vi "Run Bfr Tx - Untimed.vi"(7 "Process in":refnum<class "Process.lvclass">, 8 "error in (no error)":errorcluster, 11 "Tx Loop Data in":T1={"General Resources"={"Packet Name"="", "Packet ID"=0, "Local IP Address"="", "Local Port"=0, "Multicast"=FALSE, "Multicast IP Address"=0, "Header Info"=[], "Byte Order"=enum."big-endian, network order", "Channel Data Types"=[], "Duplex Packets"=refnum}, "Header Details"={"Packet Size"=0, "Protocol Revision"=0, "System Definition Version"=0, "Source Node Name"="", "Packet ID"=0, "Number of Channels"=0, "Static Header Size"=0, "Total Header Size"=0}, "Buffer Resources"={"Data Buffer"=0, "Pointer Encoding"=enum."Direct Encoding", "Buffer Size"=0, "Raw Buffer Data"=[], "Is Buffered"=FALSE, "External Buffer"=FALSE, "Prepend Header"=FALSE, "Valid Buffer"=FALSE}, "Runtime Resources"={"Connection ID"=refnum, "Transmit Option"=enum."Always", "Destination IP Address"=0, "Destination Port"=0, "Multicast IP Address"=0, "TTL"=0, "Multicast"=FALSE, "Port as Channel"=FALSE, "ExecutionConfig"={"Loop Period"=0, "RT Loop Period"=-2, "Untimed Period"=0, "Target Processor"=0, "Priority"=0, "Thread Management"=enum."Untimed (Default)"}}, "Echo Resources"={"Transmit Echo Option"=enum."PCL Reset", "Packet Count"=0.0, "Counter Increment"=0.0, "Transmit Values"=[]}, "Buffer Option Support"={"Buffer Option"=enum."Static Buffer", "Sim Option"=enum."No Simulation"}, "Channel Resources"={"Transmit Flag"=refnum, "Transmit Echo"=refnum, "Transmit Bytes"=refnum, "Port Channel"=refnum, "Buffer (External)"=refnum, "Buffer (Local)"=refnum, "Timestamp"=refnum}, "Debug Resources"={"Debug Mode"=FALSE, "Debug Log File"=refnum, "Packet Name"=""}} {"Buffer Resources"."Data Buffer" format="%016x"}) -> (3 "Tx Loop Data out":T1={"General Resources"={"Packet Name"="", "Packet ID"=0, "Local IP Address"="", "Local Port"=0, "Multicast"=FALSE, "Multicast IP Address"=0, "Header Info"=[], "Byte Order"=enum."big-endian, network order", "Channel Data Types"=[], "Duplex Packets"=refnum}, "Header Details"={"Packet Size"=0, "Protocol Revision"=0, "System Definition Version"=0, "Source Node Name"="", "Packet ID"=0, "Number of Channels"=0, "Static Header Size"=0, "Total Header Size"=0}, "Buffer Resources"={"Data Buffer"=0, "Pointer Encoding"=enum."Direct Encoding", "Buffer Size"=0, "Raw Buffer Data"=[], "Is Buffered"=FALSE, "External Buffer"=FALSE, "Prepend Header"=FALSE, "Valid Buffer"=FALSE}, "Runtime Resources"={"Connection ID"=refnum, "Transmit Option"=enum."Always", "Destination IP Address"=0, "Destination Port"=0, "Multicast IP Address"=0, "TTL"=0, "Multicast"=FALSE, "Port as Channel"=FALSE, "ExecutionConfig"={"Loop Period"=0, "RT Loop Period"=-2, "Untimed Period"=0, "Target Processor"=0, "Priority"=0, "Thread Management"=enum."Untimed (Default)"}}, "Echo Resources"={"Transmit Echo Option"=enum."PCL Reset", "Packet Count"=0.0, "Counter Increment"=0.0, "Transmit Values"=[]}, "Buffer Option Support"={"Buffer Option"=enum."Static Buffer", "Sim Option"=enum."No Simulation"}, "Channel Resources"={"Transmit Flag"=refnum, "Transmit Echo"=refnum, "Transmit Bytes"=refnum, "Port Channel"=refnum, "Buffer (External)"=refnum, "Buffer (Local)"=refnum, "Timestamp"=refnum}, "Debug Resources"={"Debug Mode"=FALSE, "Debug Log File"=refnum, "Packet Name"=""}} {"Buffer Resources"."Data Buffer" format="%016x"})   [LabVIEW 2016, in "UDP-Custom-Device Engine.lvlib"]
uses:
  UDP-Custom-Device Engine.lvlib
  <vilib>/NI/NIVS Inline Async API/_VS Inline Async API/Process/Process.lvclass
  Types/Engine - Buffered Tx Loop Data.ctl
  Types/Engine - General Resources.ctl
  <vilib>/NI Veristand/VeriStand Data/Typedefs/Typedefs.Data Types.ctl
  Shared/Types/Shared - Duplex Settings.ctl
  Shared/Types/Shared - Header Details.ctl
  Types/Engine - Buffer Resources.ctl
  Shared/Types/Shared - Pointer Encoding.ctl
  Types/Engine - Tx Runtime Resources.ctl
  Shared/Types/Shared - Transmit Flag Options.ctl
  Types/Engine - Execution Config.ctl
  Shared/Types/Shared - Thread Management.ctl
  Types/Engine - Tx Echo Resources.ctl
  Shared/Types/Shared - Transmit Echo Options.ctl
  Types/Engine - Buffered Tx Buffer Option Support.ctl
  Shared/Types/Shared - Transmit Buffer Options.ctl
  Shared/Types/Shared - Transmit Sim Options.ctl
  Types/Engine - Buffered Tx Channel Refs.ctl
  <vilib>/NI/NIVS Inline Async API/_Data Access Engine/Data Access Engine/Types/Read.DVR.ctl
  <vilib>/NI/NIVS Inline Async API/_Data Access Engine/Access Type Classes/Read/Read.lvclass
  <vilib>/NI/NIVS Inline Async API/_Data Access Engine/Data Access Engine/Types/Write.DVR.ctl
  <vilib>/NI/NIVS Inline Async API/_Data Access Engine/Access Type Classes/Write/Write.lvclass
  Types/Engine - Debug Resources.ctl
  <vilib>/NI/NIVS Inline Async API/_Data Access Engine/Access Type Classes/Read/Read.lvclass/Read.ctl
  <vilib>/NI/NIVS Inline Async API/_Data Access Engine/Access Type Classes/Write/Write.lvclass/Write.ctl
  <vilib>/NI/NIVS Inline Async API/_VS Inline Async API/Process/Process.lvclass/Process.ctl
  <vilib>/NI Veristand/VeriStand Data/Pointer Operations/Pointer.Write.vi
  <vilib>/NI Veristand/VeriStand Data/Pointer Operations/Pointer.Write (String).vi
  <vilib>/NI Veristand/VeriStand Data/Pointer Operations/Pointer.Write (1D U8).vi
  <vilib>/NI Veristand/VeriStand Data/Pointer Operations/Pointer.Write (I32).vi
  <vilib>/NI Veristand/VeriStand Data/Pointer Operations/Pointer.Write (U16).vi
  <vilib>/NI/NIVS Inline Async API/_Data Access Engine/Data Access Engine/Methods/Data.Processes.Execute.vi
  <vilib>/NI/NIVS Inline Async API/_Data Access Engine/Data Access Engine/Methods/Read.Data.vi
  Transmit/Run Tx - Handle Transmit Option.vi
  Run Bfr Tx - Handle Transmit Size.vi
  Transmit/Run Tx - Handle Port Tx Check.vi
  <vilib>/NI/NIVS Inline Async API/_Data Access Engine/Data Access Engine/Methods/Write.Data.vi
  <vilib>/NI Veristand/VeriStand Data/Pointer Operations/Pointer.In-Place Read.vi
  <vilib>/NI Veristand/VeriStand Data/Pointer Operations/Pointer.In-Place Read (1D U8).vi
  Run Bfr Tx - FIFO Entry Size.vi
  Run Bfr Tx - FIFO Payload.vi
  Run Bfr Tx - FIFO Count Packets.vi
  Run Bfr Tx - FIFO Port.vi
  <vilib>/NI/NIVS Inline Async API/_VS Inline Async API/Error Handling Process/SubVIs/Error.ConvertArray.vi
  <vilib>/NI/NIVS Inline Async API/_Data Access Engine/Access Type Classes/Read/Read.ProcessData.vi
  <vilib>/NI Veristand/VeriStand Data/Type Conversion/Type Conversion.From Double.vi
  <vilib>/NI Veristand/VeriStand Data/Type Conversion/Type Conversion.From Double (I32).vi
  <vilib>/NI/NIVS Inline Async API/_Data Access Engine/Access Type Classes/Write/Write.ProcessData.vi
  <vilib>/NI Veristand/VeriStand Data/Pointer Operations/Pointer.Read.vi
  <vilib>/NI Veristand/VeriStand Data/Pointer Operations/Pointer.Read (I32).vi
  <vilib>/NI Veristand/VeriStand Data/Pointer Operations/Pointer.Read (U16).vi
  <vilib>/NI Veristand/VeriStand Data/Pointer Operations/Pointer.In-Place Read (I32).vi
  <vilib>/NI Veristand/VeriStand Data/Pointer Operations/Pointer.In-Place Read (U16).vi
  <vilib>/NI Veristand/VeriStand Data/VeriStand Data.lvlib
  Shared/UDP-Custom-Device Shared.lvlib
  <vilib>/NI/NIVS Inline Async API/_Data Access Engine/Data Access Engine/Data Access Engine.lvclass
panel:
  out "dataBuffer":u64 format="%016x"
  out "Tx Packet":string
  # "BUFFERED TRANSMIT\n- UNTIMED\n- ALL TARGETS"
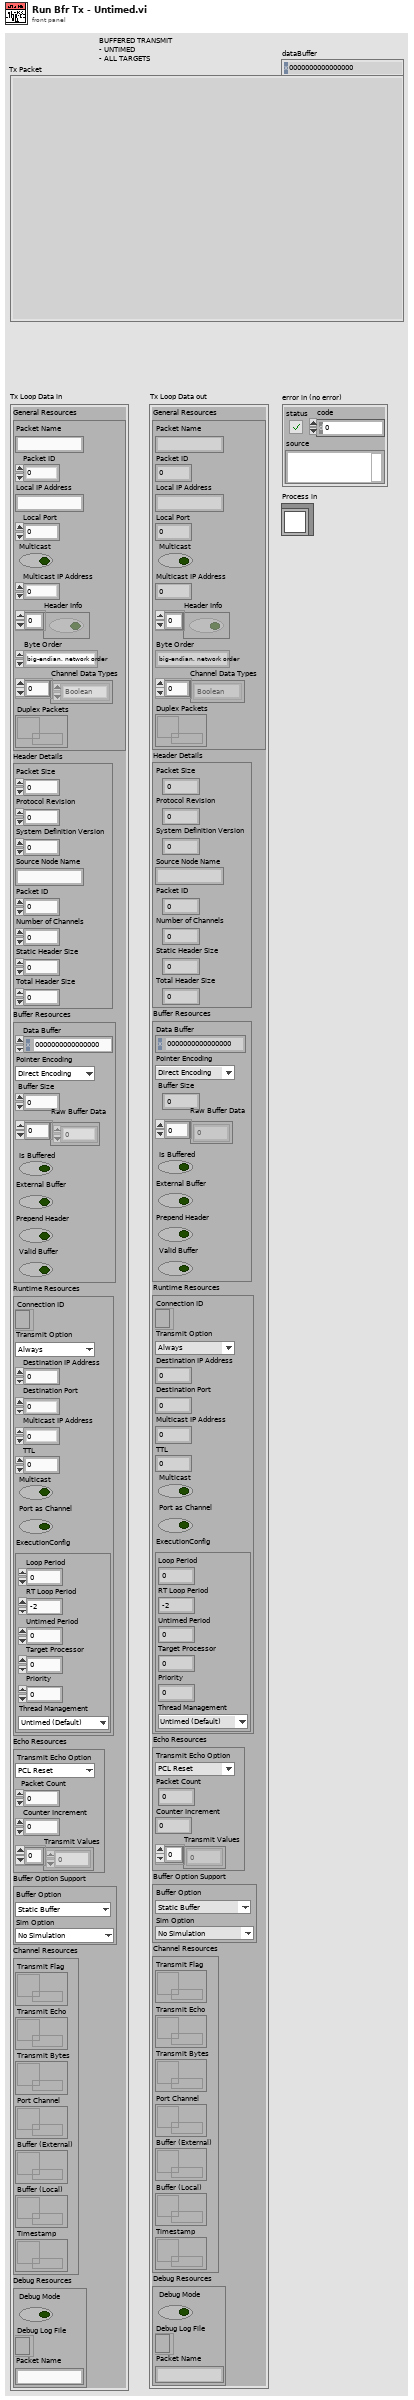
[diagram p1: front panel]
types:
  T1 = typedef "UDP-Custom-Device Engine.lvlib/Engine - Buffered Tx Loop Data.ctl" = cluster{"General Resources":T2, "Header Details":T4, "Buffer Resources":T5, "Runtime Resources":T7, "Echo Resources":T11, "Buffer Option Support":T13, "Channel Resources":T16, "Debug Resources":T19}
  T2 = typedef "UDP-Custom-Device Engine.lvlib/Engine - General Resources.ctl" = cluster{"Packet Name":string, "Packet ID":i32, "Local IP Address":string, "Local Port":i32, "Multicast":bool, "Multicast IP Address":u32, "Header Info":bool[], "Byte Order":enum16{"big-endian, network order", "native, host order", "little-endian"}, "Channel Data Types":T3[], "Duplex Packets":refnum<data-value>}
  T3 = typedef "VeriStand Data.lvlib/Typedefs.Data Types.ctl" = enum16{"Boolean", "Single", "Double", "I8", "I16", "I32", "I64", "U8", "U16", "U32", "U64"}
  T4 = typedef "UDP-Custom-Device Shared.lvlib/Shared - Header Details.ctl" = cluster{"Packet Size":u16, "Protocol Revision":u8, "System Definition Version":u64, "Source Node Name":string, "Packet ID":u32, "Number of Channels":u32, "Static Header Size":u16, "Total Header Size":u16}
  T5 = typedef "UDP-Custom-Device Engine.lvlib/Engine - Buffer Resources.ctl" = cluster{"Data Buffer":u64, "Pointer Encoding":T6, "Buffer Size":u64, "Raw Buffer Data":u8[], "Is Buffered":bool, "External Buffer":bool, "Prepend Header":bool, "Valid Buffer":bool}
  T6 = typedef "UDP-Custom-Device Shared.lvlib/Shared - Pointer Encoding.ctl" = enum16{"Direct Encoding", "Conversion Encoding"}
  T7 = typedef "UDP-Custom-Device Engine.lvlib/Engine - Tx Runtime Resources.ctl" = cluster{"Connection ID":refnum<k16>, "Transmit Option":T8, "Destination IP Address":u32, "Destination Port":u16, "Multicast IP Address":u32, "TTL":u16, "Multicast":bool, "Port as Channel":bool, "ExecutionConfig":T9}
  T8 = typedef "UDP-Custom-Device Shared.lvlib/Shared - Transmit Flag Options.ctl" = enum16{"Always", "One-Shot", "Toggle"}
  T9 = typedef "UDP-Custom-Device Engine.lvlib/Engine - Execution Config.ctl" = cluster{"Loop Period":i64, "RT Loop Period":i64, "Untimed Period":u32, "Target Processor":i32, "Priority":i32, "Thread Management":T10}
  T10 = typedef "UDP-Custom-Device Shared.lvlib/Shared - Thread Management.ctl" = enum16{"Untimed (Default)", "Timed (High Priority)"}
  T11 = typedef "UDP-Custom-Device Engine.lvlib/Engine - Tx Echo Resources.ctl" = cluster{"Transmit Echo Option":T12, "Packet Count":dbl, "Counter Increment":dbl, "Transmit Values":dbl[]}
  T12 = typedef "UDP-Custom-Device Shared.lvlib/Shared - Transmit Echo Options.ctl" = enum16{"PCL Reset", "Counter", "Mirror"}
  T13 = typedef "UDP-Custom-Device Engine.lvlib/Engine - Buffered Tx Buffer Option Support.ctl" = cluster{"Buffer Option":T14, "Sim Option":T15}
  T14 = typedef "UDP-Custom-Device Shared.lvlib/Shared - Transmit Buffer Options.ctl" = enum16{"Static Buffer", "FIFO Buffer", "FIFO Buffer + Port"}
  T15 = typedef "UDP-Custom-Device Shared.lvlib/Shared - Transmit Sim Options.ctl" = enum16{"No Simulation", "Counter", "Full Buffer", "FIFO Test", "FIFO + Port Test"}
  T16 = typedef "UDP-Custom-Device Engine.lvlib/Engine - Buffered Tx Channel Refs.ctl" = cluster{"Transmit Flag":T17, "Transmit Echo":T18, "Transmit Bytes":T17, "Port Channel":T17, "Buffer (External)":T17, "Buffer (Local)":T18, "Timestamp":T17}
  T17 = typedef "Data Access Engine.lvlib/Data Access Engine.lvclass/Read.DVR.ctl" = refnum<data-value>
  T18 = typedef "Data Access Engine.lvlib/Data Access Engine.lvclass/Write.DVR.ctl" = refnum<data-value>
  T19 = typedef "UDP-Custom-Device Engine.lvlib/Engine - Debug Resources.ctl" = cluster{"Debug Mode":bool, "Debug Log File":refnum<file>, "Packet Name":string}
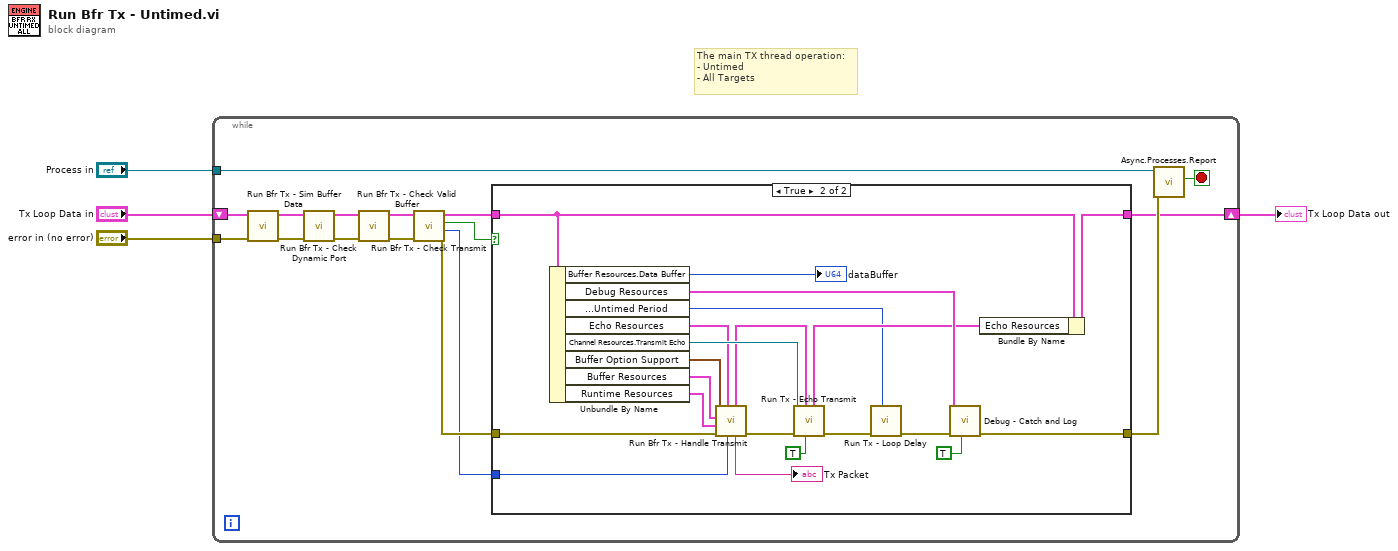
[diagram p0: block diagram]
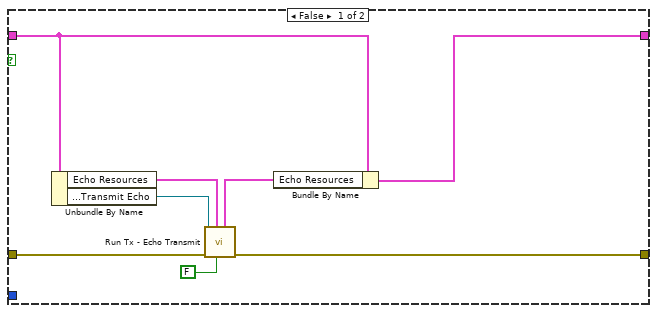
[diagram p2: hidden frame]
diagram:
  # "The main TX thread operation:\n- Untimed\n- All Targets"
  n1 = while {
    tunnel: "error in (no error)" -> [w16]
    tunnel: "Process in" -> [w20]
    shift-right: [w15] -> w1
    shift-left: "Tx Loop Data in" -> [w17]
    stop <- w19 stop-if-true
    n2 = call "Run Bfr Tx - Sim Buffer Data.vi"("error in (no error)"=w16, "Tx Loop Data in"=w17) -> ("error out"=w6:errorcluster, "Tx Loop Data out"=w8:T1)  [unwired: 8 in]
    n3 = call "Run Bfr Tx - Check Dynamic Port.vi"("error in (no error)"=w6, "Tx Loop Data in"=w8) -> ("error out"=w5:errorcluster, "Tx Loop Data out"=w7:T1)  [unwired: 8 in]
    n4 = call "Run Bfr Tx - Check Valid Buffer.vi"("error in (no error)"=w5, "Tx Loop Data in"=w7) -> ("error out"=w9:errorcluster, "Tx Loop Data out"=w10:T1)  [unwired: 8 in]
    n5 = call "Run Bfr Tx - Check Transmit.vi"("error in (no error)"=w9, "Tx Loop Data in"=w10) -> ("error out"=w14:errorcluster, "Bytes to Transmit"=w11:i32, "Transmit?"=w13:bool, "Tx Loop Data out"=w12:T1)  [unwired: 6 in]
    n6 = case shown="True" w13 {
      tunnel: [w21 w44] -> w18
      tunnel: [w24 w46] -> w15
      tunnel: w14 -> [w27 w41]
      tunnel: w12 -> [w25 w47]
      tunnel: w11 -> [_ w39]
      frame False {
        n7 = Unbundle By Name(w25) -> ("Echo Resources"=w23:T11, "Channel Resources.Transmit Echo"=w28:T18)
        n8 = call "Run Tx - Echo Transmit.vi"("Transmitted?"=FALSE, "Echo Resources in"=w23, "error in (no error)"=w27, "Ref"=w28) -> ("error out"=w21:errorcluster, "Echo Resources out"=w22:T11)  [unwired: 6 in]
        n9 = Bundle By Name(cluster=w25, "Echo Resources"=w22) -> (w24:T1)
      }
      frame True {
        n10 = Unbundle By Name(w47) -> ("Buffer Resources.Data Buffer"=→"dataBuffer":u64, "Debug Resources"=w43:T19, "Runtime Resources.ExecutionConfig.Untimed Period"=w29:u32, "Echo Resources"=w35:T11, "Channel Resources.Transmit Echo"=w49:T18, "Buffer Option Support"=w36:T13, "Buffer Resources"=w37:T5, "Runtime Resources"=w38:T7)
        n11 = call "Run Bfr Tx - Handle Transmit.vi"("Bytes to Transmit"=w39, "Echo Resources in"=w35, "error in (no error)"=w41, "Runtime Resources"=w38, "Buffer Resources"=w37, "Buffer Option Support in"=w36) -> ("error out"=w40:errorcluster, "Tx Packet"=→"Tx Packet":string, "Echo Resources out"=w34:T11)  [unwired: 3 in]
        n12 = call "Run Tx - Echo Transmit.vi"("Transmitted?"=TRUE, "Echo Resources in"=w34, "error in (no error)"=w40, "Ref"=w49) -> ("error out"=w31:errorcluster, "Echo Resources out"=w42:T11)  [unwired: 6 in]
        n13 = call "Run Tx - Loop Delay.vi"("Delay (ms)"=w29, "error in (no error)"=w31) -> ("error out"=w30:errorcluster)  [unwired: 9 in]
        n14 = call "Debug - Catch and Log.vi"("Clear Error?"=TRUE, "error in (no error)"=w30, "Debug Resources"=w43) -> ("error out"=w44:errorcluster)  [unwired: 8 in]
        n15 = Bundle By Name(cluster=w47, "Echo Resources"=w42) -> (w46:T1)
      }
    }
    n16 = call <vilib>:"Async.Processes.Report.vi"("Error"=w18, "Process in"=w20) -> ("Stop"=w19:bool)  [unwired: 8 in, 1 out]
  }
  "Tx Loop Data out" <- w1
